vi "SIP Swing-Up Control.vi"() -> ()   [LabVIEW 2013]
uses:
  <vilib>/Simulation/Scripting/Companion Diagram/SimConfigNode/SimParams.ctl
  <vilib>/Simulation/Scripting/Companion Diagram/SimConfigNode/_simSolvers.ctl
  <vilib>/Simulation/Implementation/Shared/SIMSCR Execution Mode.ctl
  <vilib>/Platform/TimedLoop/XDataNode/timing_clust.ctl
  <vilib>/Platform/TimedLoop/XDataNode/nitl_modes.ctl
  <vilib>/Platform/TimedLoop/XDataNode/wakeup.ctl
  <vilib>/Simulation/Param Hierarchy/Typedefs/SIMPH Param Control Actions.ctl
  <vilib>/Simulation/Implementation/Shared/NILVSim_ParamChanged.vi
  <vilib>/Simulation/Implementation/Shared/NILVSim_FinishedLate.vi
  <vilib>/Simulation/Implementation/Shared/NILVSIM_BeginStep.vi
  <vilib>/Simulation/DataSources/Implementation/NILVSim Signal Generator.llb/SIM Signal Generator (scalar).vi
  <vilib>/Simulation/SignalArithmetic/Implementation/NILVSim Gain.llb/SIM Gain (scalar).vi
  <vilib>/Simulation/Utility/Implementation/SIM Halt.vi
  <vilib>/Simulation/SignalArithmetic/Implementation/NILVSim Gain.llb/SIM Gain (vector).vi
  <vilib>/Simulation/Utility/Implementation/NILVSim Memory.llb/NILVSim Memory (core).vi
  <vilib>/Simulation/ContinuousLinear/Implementation/NILVSim Transfer Function.llb/SIM Transfer Function Distributor (SISO).vi
  <vilib>/Simulation/ContinuousLinear/Implementation/NILVSim Transfer Function.llb/SIM Transfer Function Collector (SISO).vi
  <vilib>/Simulation/Nonlinear/Implementation/NILVSim Saturation.llb/SIM Saturation (scalar).vi
  <vilib>/Simulation/SignalArithmetic/Implementation/NILVSim Gain.llb/SIM Gain (vector,MatrixGain).vi
  <vilib>/Simulation/Implementation/Shared/NILVSim_Manager.vi
  <vilib>/Simulation/Implementation/Shared/NILVSim_FinalizeModel.vi
  <vilib>/Simulation/Implementation/Shared/SIM Unbundle Sim Info.vi
  <vilib>/Utility/error.llb/Clear Errors.vi
  <vilib>/Simulation/Implementation/Shared/NILVSim_GetModelError.vi
  <vilib>/Simulation/Implementation/Shared/SIM Bundle Sim Info.vi
  <vilib>/Simulation/Implementation/Shared/SIMSH Read Queue.vi
  <vilib>/Simulation/Implementation/Shared/NILVSim_Initialize.vi
  <vilib>/Simulation/Utility/Implementation/NILVSim Get Time and IsAcceptedStep.vi
  <vilib>/Simulation/Scripting/Companion Diagram/SimConfigNode/SimDog.xnode
  <vilib>/Quanser/Rapid Control Prototyping Toolkit/hardware/HIL Immediate IO/_TypeSpecific/CL HIL Write Analog (Scalar).vi
  <vilib>/Quanser/Rapid Control Prototyping Toolkit/hardware/HIL Immediate IO/CL HIL Write.vi
  <vilib>/Quanser/Rapid Control Prototyping Toolkit/hardware/HIL Immediate IO/_TypeSpecific/CL HIL Read Encoder (Vector).vi
  <vilib>/Quanser/Rapid Control Prototyping Toolkit/hardware/HIL Immediate IO/CL HIL Read.vi
  <vilib>/Platform/TimedLoop/XDataNode/XDataNode.xnode
  <vilib>/Simulation/Implementation/XNodeFramework/SimXNode/SimX.xnode
  <vilib>/Simulation/ContinuousLinear/Implementation/NILVSim Transfer Function.llb/SIM Transfer Function (SISO).vi
  <vilib>/Simulation/Implementation/Shared/NI_SIM_Implementation.lvlib
  <vilib>/Platform/TimedLoop/XDataNode/XDNodeRunTimeDep.lvlib
panel:
  in  "Km":dbl=0.0077
  in  "Kt":dbl=0.0077
  in  "Kg":dbl=3.71
  in  "r_mp":dbl=0.0063
  in  "Rm":dbl=2.6
  in  "Mc":dbl=1.0731
  out "Pendulum Energy (J)":dbl
  in  "u_max (m/s^2)":dbl=1.0
  in  "mu":dbl
  in  "Er (J)":dbl=1.49
  in  "Jp":dbl=0.0079
  in  "lp":dbl=0.3302
  in  "Mp":dbl=0.23
  out "Motor Voltage (V)":dbl(graph)
  in  "Setpoint Amplitude (mm)":dbl
  out "In Range?":bool=TRUE
  in  "Feedback Gain":dbl[][](array[numeric])=[[-30.0, 150.0, -40.0, 20.0]]
  out "Pendulum Angle (deg)":dbl(graph)
  out "Cart Position (mm)":cluster{"output":dbl, "output":dbl}(graph)
  in  "Stop Button":bool
  # "Control Parameters"
  # "Pendulum Parameters"
  # "IP02 Cart Parameters"
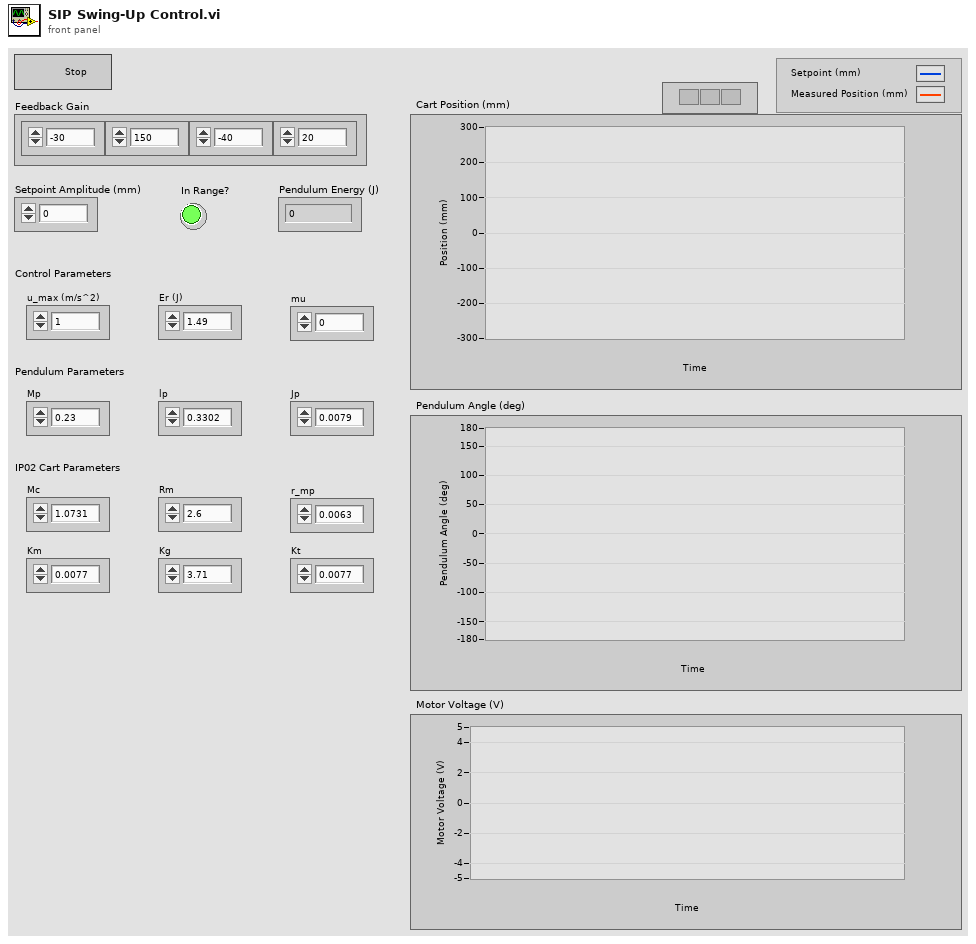
[diagram p1: front panel]
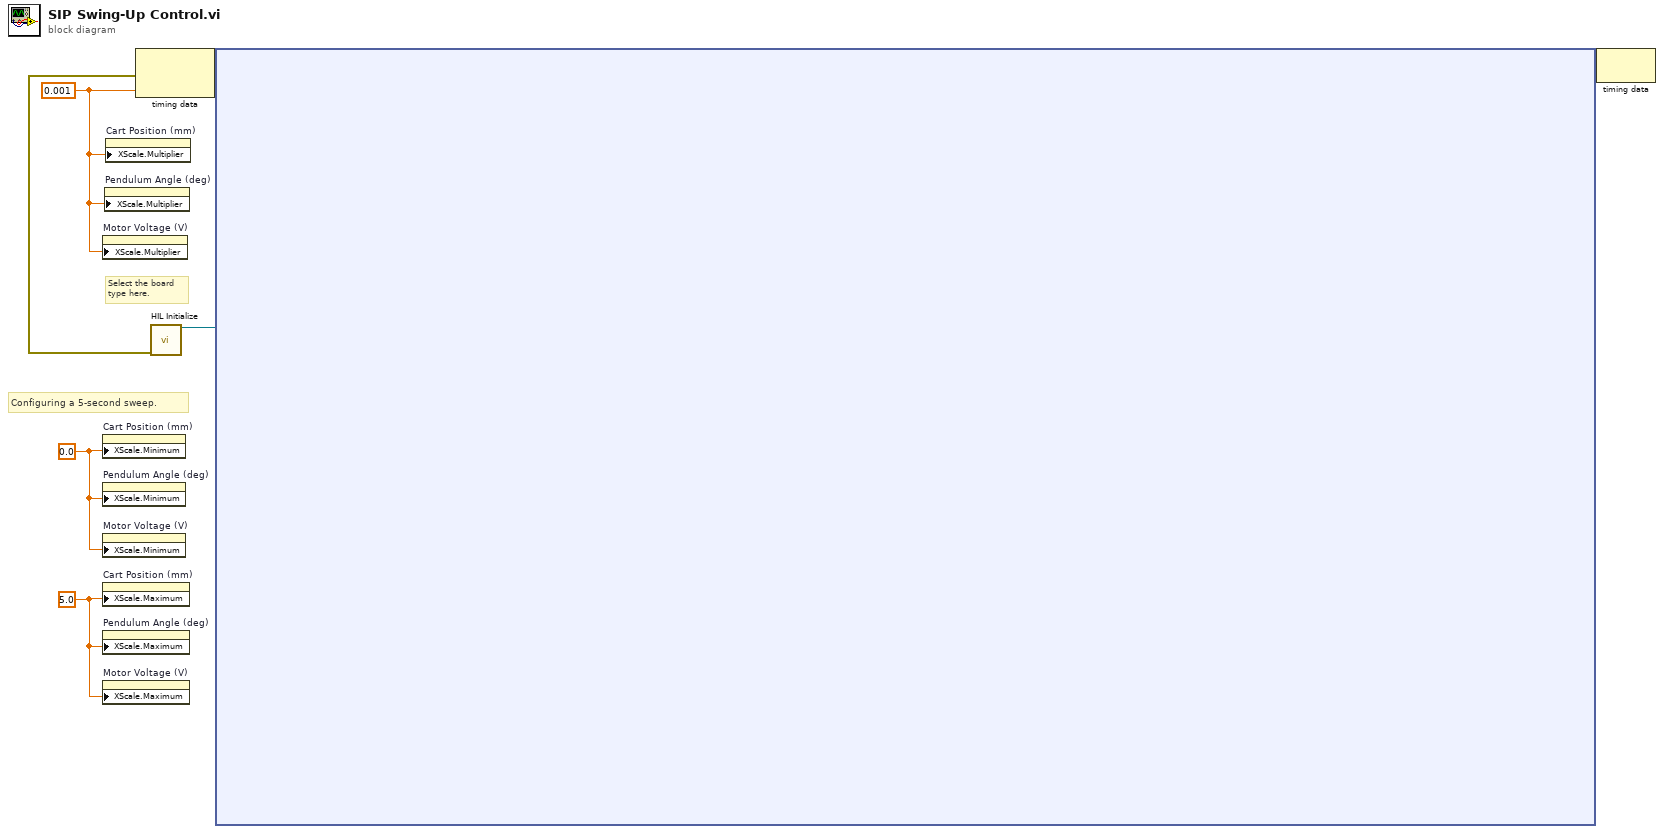
[diagram p0: block diagram]
diagram:
  w2 = 0.0 ("X Scale.Range:Minimum")
  w1 = 5.0 ("X Scale.Range:Maximum")
  w3 = 0.001 ("Step Size (s)")
  # "Configuring a 5-second sweep."
  # "Select the board\ntype here."
  n1 = property on="Motor Voltage (V)" class="WFChart (strict)"("XScale.Multiplier"=w3) -> ()  [unwired: 2 in, 2 out]
  n2 = property on="Cart Position (mm)" class="WFChart (strict)"("XScale.Minimum"=w2) -> ()  [unwired: 2 in, 2 out]
  n3 = property on="Pendulum Angle (deg)" class="WFChart (strict)"("XScale.Minimum"=w2) -> ()  [unwired: 2 in, 2 out]
  n4 = property on="Motor Voltage (V)" class="WFChart (strict)"("XScale.Minimum"=w2) -> ()  [unwired: 2 in, 2 out]
  n5 = property on="Cart Position (mm)" class="WFChart (strict)"("XScale.Maximum"=w1) -> ()  [unwired: 2 in, 2 out]
  n6 = property on="Pendulum Angle (deg)" class="WFChart (strict)"("XScale.Maximum"=w1) -> ()  [unwired: 2 in, 2 out]
  n7 = property on="Motor Voltage (V)" class="WFChart (strict)"("XScale.Maximum"=w1) -> ()  [unwired: 2 in, 2 out]
  n8 = property on="Pendulum Angle (deg)" class="WFChart (strict)"("XScale.Multiplier"=w3) -> ()  [unwired: 2 in, 2 out]
  n9 = property on="Cart Position (mm)" class="WFChart (strict)"("XScale.Multiplier"=w3) -> ()  [unwired: 2 in, 2 out]
  n10 = call "HIL Initialize"() -> ("board out"=w5:refnum<class "HIL Board.lvclass">, "error out"=w4:errorcluster)  [unwired: 14 in]
  n11 = node-c288(w4, w3) -> (w7:variant)
  n12 = node-c254 ("Control & Simulation Loop")(w7, w5) -> (w6:variant)
  n13 = node-c288(w6) -> ()  [unwired: 1 out]
